vi "get debug info.vi"(0 "core_data":T2) -> ()   [LabVIEW 2020, in "core.lvlib"]
uses:
  core.lvlib
  core_data/core_data.ctl
  core_data/tour_in_progress.ctl
  core_data/chessboard_index.ctl
  core_data/chess_square.ctl
  core_data/neighbour_square.ctl
  core_data/core_data.lvlib
panel:
  out "CurrentTour Count":i32
  out "CurrentTour":T1[](array[typedef])
  out "Indexes of exhausted neighbours":i32[](array[numeric])
  out "Contain exhausted neighbours":T1[](array[typedef])
  out "Unexplored squares":T1[](array[typedef])
  out "no of Exhausted neighbours":i32
  out "no of Explored squares":i32
  out "total no. of moves backward":u64
  out "total no. of moves forward":u64
  # "Development\ncontrols/indicators useful for development and testing, but which are not outputs of the VI"
  # "Input\nInputs to the VI"
  # "Output\nOutputs of the VI"
  # "Description\n\nBlank VI with error handling case. \n\nSummarize the use of this VI in this space."
  # "Explored"
  # "Exhausted"
  # "Current Tour"
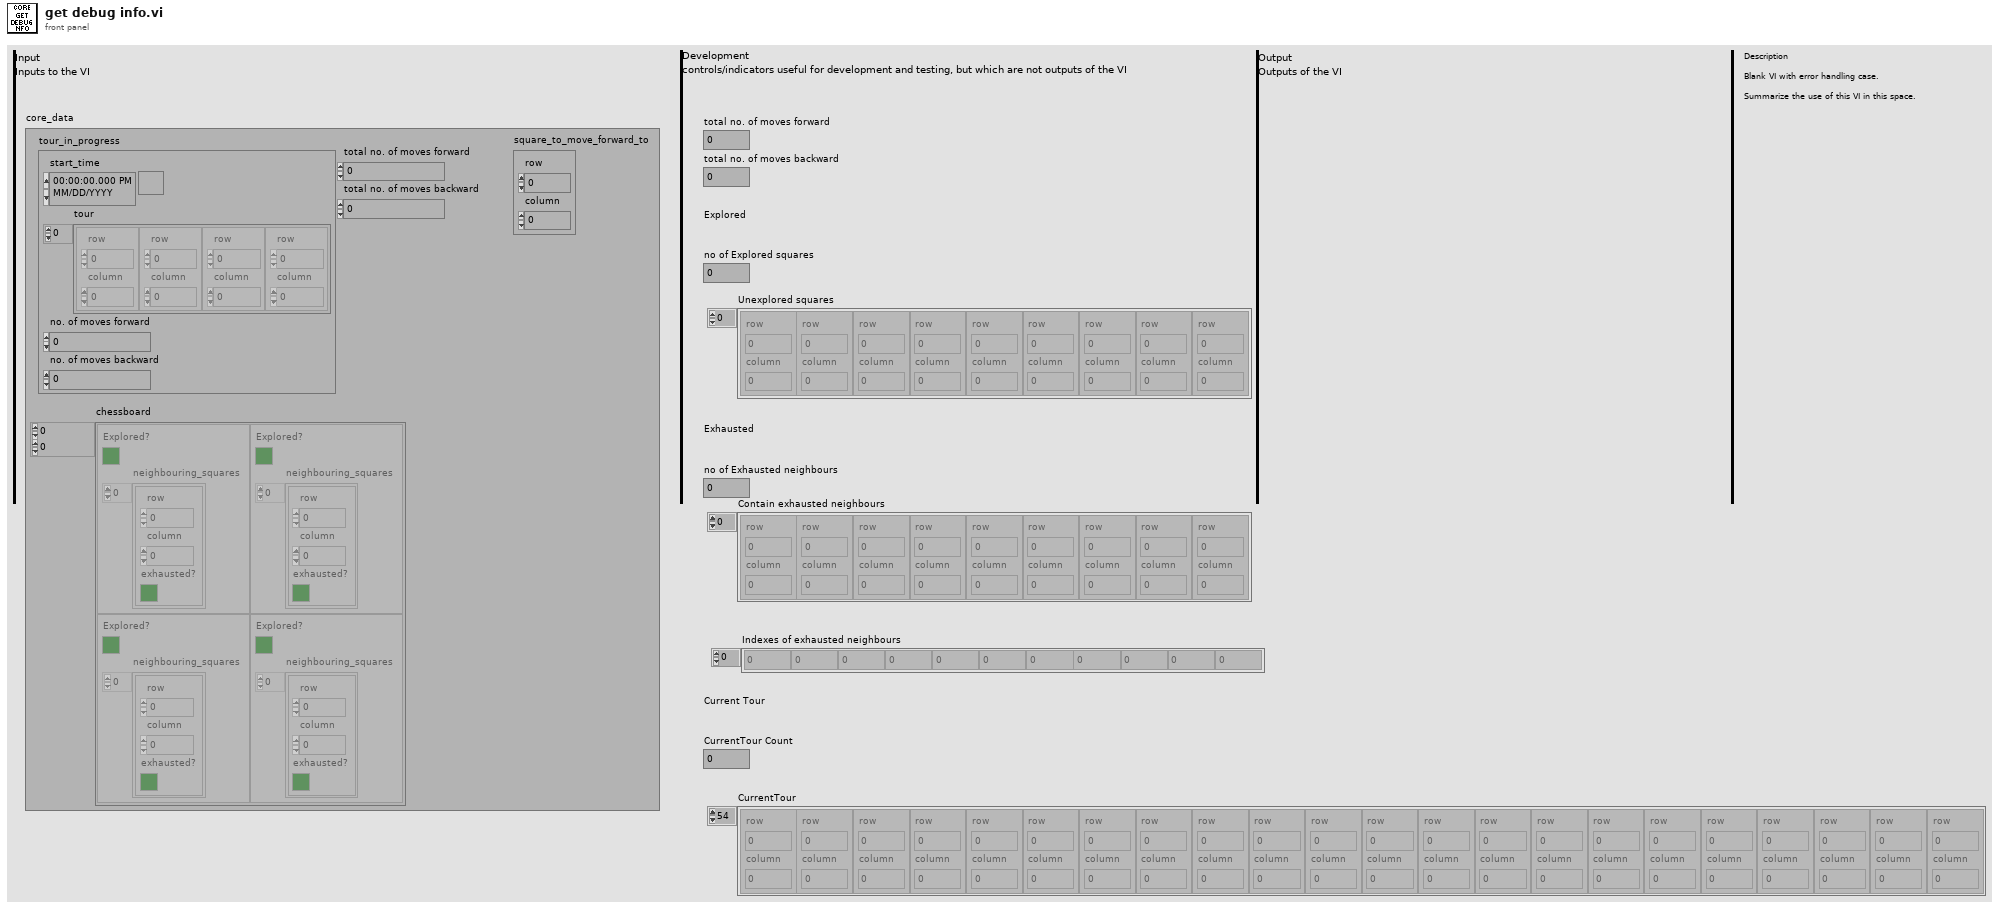
[diagram p1: front panel]
types:
  T1 = typedef "core.lvlib/core_data.lvlib/chessboard_index.ctl" = cluster{"row":u8, "column":u8}
  T2 = typedef "core.lvlib/core_data.lvlib/core_data.ctl" = cluster{"tour_in_progress":T3, "total no. of moves forward":u64, "total no. of moves backward":u64, "chessboard":T4[][], "square_to_move_forward_to":T1}
  T3 = typedef "core.lvlib/core_data.lvlib/tour_in_progress.ctl" = cluster{"start_time":timestamp, "tour":T1[], "no. of moves forward":u64, "no. of moves backward":u64}
  T4 = typedef "core.lvlib/core_data.lvlib/chess_square.ctl" = cluster{"Explored?":bool, "neighbouring_squares":T5[]}
  T5 = typedef "core.lvlib/core_data.lvlib/neighbour_square.ctl" = cluster{"row":u8, "column":u8, "exhausted?":bool}
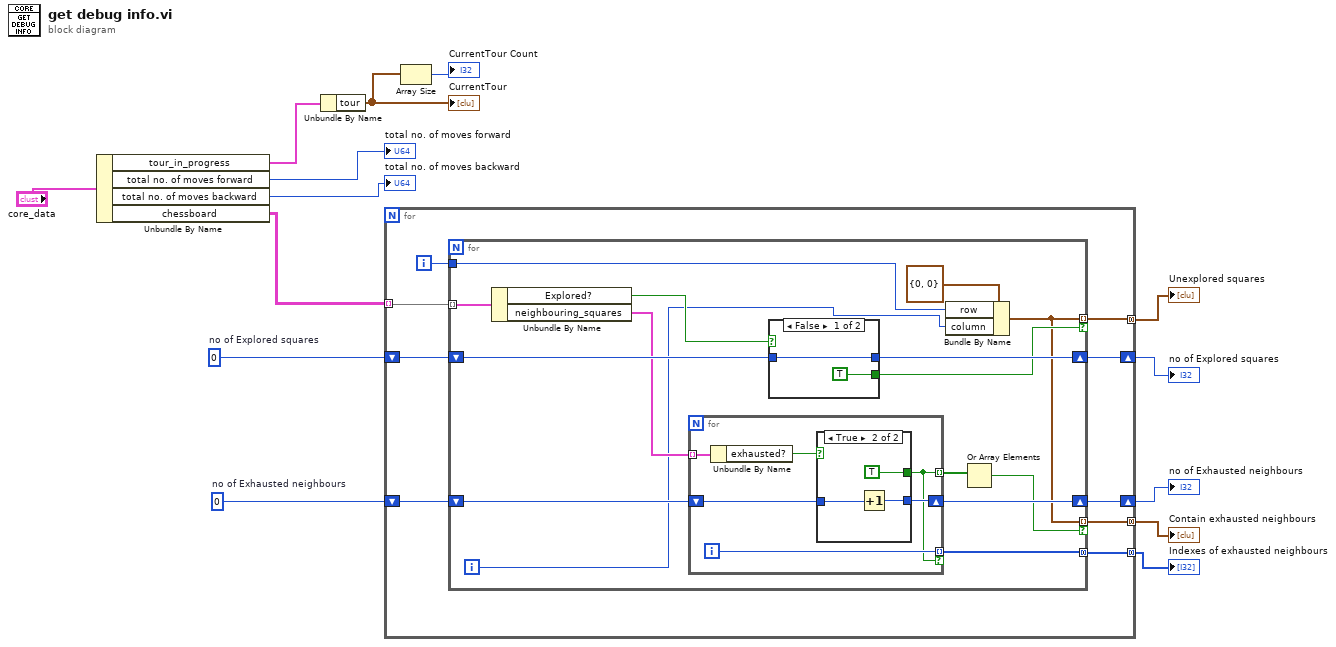
[diagram p0: block diagram]
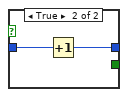
[diagram p3: hidden frame]
diagram:
  w8 = 0  # no of Exhausted neighbours
  w10 = 0  # no of Explored squares
  n1 = Unbundle By Name("core_data") -> ("tour_in_progress"=w3:T3, "total no. of moves forward"=→"total no. of moves forward":u64, "total no. of moves backward"=→"total no. of moves backward":u64, "chessboard"=w11:T4[][])
  n2 = Unbundle By Name(w3) -> ("tour"=w2:T1[])
  "CurrentTour" <- w2
  n3 = for {
    tunnel: w11 -> [w23] mode=indexing
    shift-right: [w21] -> w9
    shift-left: w10 -> [w22]
    shift-right: [w19] -> w7
    shift-left: w8 -> [w20]
    tunnel: [w17] -> w6 mode=concatenating
    tunnel: [w16] -> w5 mode=concatenating
    tunnel: [w15] -> w4 mode=concatenating
    i -> [w18]
    n4 = for {
      tunnel: w23 -> [w38] mode=indexing
      shift-right: [w35] -> w21
      shift-left: w22 -> [w36]
      shift-right: [w32] -> w19
      shift-left: w20 -> [w33]
      tunnel: w18 -> [w30]
      tunnel: [w27] -> w17 mode=indexing if=w28
      tunnel: [w27] -> w16 mode=indexing if=w25
      tunnel: [w24] -> w15 mode=concatenating
      i -> [w29]
      n5 = Unbundle By Name(w38) -> ("Explored?"=w37:bool, "neighbouring_squares"=w34:T5[])
      n6 = for {
        tunnel: w34 -> [w44] mode=indexing
        shift-right: [w41] -> w32
        shift-left: w33 -> [w42]
        tunnel: [w39] -> w26 mode=indexing
        tunnel: [w40] -> w24 mode=indexing if=w39
        i -> [w40]
        n7 = Unbundle By Name(w44) -> ("exhausted?"=w43:bool)
        n8 = case shown="True" w43 {
          tunnel: w42 -> [w45 w48]
          tunnel: [w45 w47] -> w41
          tunnel: [_ TRUE] -> w39
          frame False {
          }
          frame True {
            n9 = Increment(x=w48) -> (x+1=w47:i32)
          }
        }
      }
      n10 = case shown="False" w37 {
        tunnel: w36 -> [w50 w52]
        tunnel: [w50 w51] -> w35
        tunnel: [TRUE _] -> w28
        frame False {
        }
        frame True {
          n11 = Increment(x=w52) -> (x+1=w51:i32)
        }
      }
      n12 = Bundle By Name(cluster=T1 {"row"=0, "column"=0} ("chessboard_index"), "row"=w30, "column"=w29) -> (w27:T1)
      n13 = Or Array Elements(Boolean array=w26) -> (logical OR=w25:bool)
    }
  }
  "no of Explored squares" <- w9
  "no of Exhausted neighbours" <- w7
  "Unexplored squares" <- w6
  "Contain exhausted neighbours" <- w5
  "Indexes of exhausted neighbours" <- w4
  n14 = Array Size(array=w2) -> (size(s)=→"CurrentTour Count":i32)
